vi "CRYGraph Set.vi"(9 "Title State":bool, 10 "Graph Property":T2, 11 "pGraph VI In":refnum<vi>) -> ()   [LabVIEW 2013]
uses:
  Control/CRYPolar Property.ctl
  Control/CRYTable Property.ctl
  Control/CRYGraph Property.ctl
  Control/CRYResult Property.ctl
panel:
  in  "Result Property":T1={"Show Limits"=FALSE, "Show Yield"=FALSE, "Pass/Fail"=FALSE, "Notation"=0, "Digits"=0, "Precision"=0, "Hide Traling Zeros"=FALSE, "Show vertical scroll bar"=FALSE, "Show horizontal scroll bar"=FALSE, "True"="NO ELECTRICAL SIGNAL DETECTED!\nCheck wiring and connections.", "False"="NO ELECTRICAL SIGNAL DETECTED!\nCheck wiring and connections.", "Font Size"=0, "Overall/Optional"=0} {"Precision" items=["Digits of precision", "Significant digits"]}
  in  "Table Property":T3 {"Precision" items=["Digits of precision", "Significant digits"]}
  in  "Polar Property":T4={"polar attributes"={"maximum"=2.0, "minimum"=0.0, "clip to min"=FALSE, "log"=FALSE, "grid color"=3381657, "plot color"=16711680, "fmt and prec"={"format"=enum."Decimal", "precision"=2}, "visible section"=4}, "Auto/Manual"=0, "Zero Adjust (deg)"=0, "Angle Increment (deg)"=0, "Mirror"=FALSE, "Auto Increment"=FALSE, "Total Rotatin (deg)"=0, "Discrete/Rannge"=0, "Show Name"=FALSE, "CurValues"=[], "CurIndex"=0, "CurColors"=[], "CurColors_Range"=[], "CurValues_Range"=[], "Pen"={"Width"=1, "Style"=enum."Solid"}, "BackgroundColor"=0} {"polar attributes"."minimum" format="%0.2f"; "polar attributes"."maximum" format="%0.2f"}
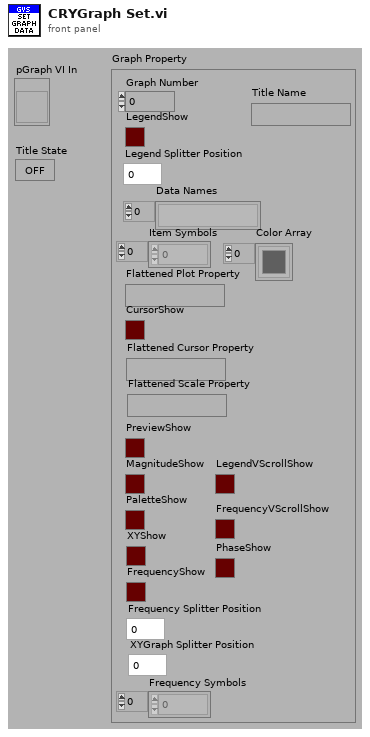
[diagram p1: front panel]
types:
  T1 = typedef "CRYResult Property.ctl" = cluster{"Show Limits":bool, "Show Yield":bool, "Pass/Fail":bool, "Notation":u16, "Digits":u16, "Precision":u16, "Hide Traling Zeros":bool, "Show vertical scroll bar":bool, "Show horizontal scroll bar":bool, "True":string, "False":string, "Font Size":u16, "Overall/Optional":u16}
  T2 = typedef "CRYGraph Property.ctl" = cluster{"LegendShow":bool, "Legend Splitter Position":dbl, "Data Names":string[], "Item Symbols":i32[], "Color Array":u32[], "Flattened Plot Property":string, "CursorShow":bool, "Flattened Cursor Property":string, "Graph Number":i32, "Flattened Scale Property":string, "PreviewShow":bool, "MagnitudeShow":bool, "PaletteShow":bool, "XYShow":bool, "FrequencyShow":bool, "Frequency Splitter Position":dbl, "XYGraph Splitter Position":dbl, "Frequency Symbols":i32[], "LegendVScrollShow":bool, "FrequencyVScrollShow":bool, "PhaseShow":bool, "Title Name":string}
  T3 = typedef "CRYTable Property.ctl" = cluster{"Reset All Columns":bool, "Transpose":bool, "Display Units":bool, "Notation":u16, "Digits":u16, "Precision":u16, "Hide Traling Zeros":bool, "Column Width":u16, "Row Header Width":u16, "Show vertical scroll bar":bool, "Show horizontal scroll bar":bool}
  T4 = typedef "CRYPolar Property.ctl" = cluster{"polar attributes":cluster{"maximum":dbl, "minimum":dbl, "clip to min":bool, "log":bool, "grid color":u32, "plot color":u32, "fmt and prec":cluster{"format":enum8{"Decimal", "Scientific", "Engineering", "Binary", "Octal", "Hex"}, "precision":u8}, "visible section":u16}, "Auto/Manual":u16, "Zero Adjust (deg)":i32, "Angle Increment (deg)":i32, "Mirror":bool, "Auto Increment":bool, "Total Rotatin (deg)":i32, "Discrete/Rannge":u16, "Show Name":bool, "CurValues":dbl[], "CurIndex":u16, "CurColors":u32[], "CurColors_Range":u32[], "CurValues_Range":dbl[], "Pen":cluster{"Width":u16, "Style":enum32{"Solid", "Dash", "Dot", "DashDot", "DashDotDot"}}, "BackgroundColor":u32}
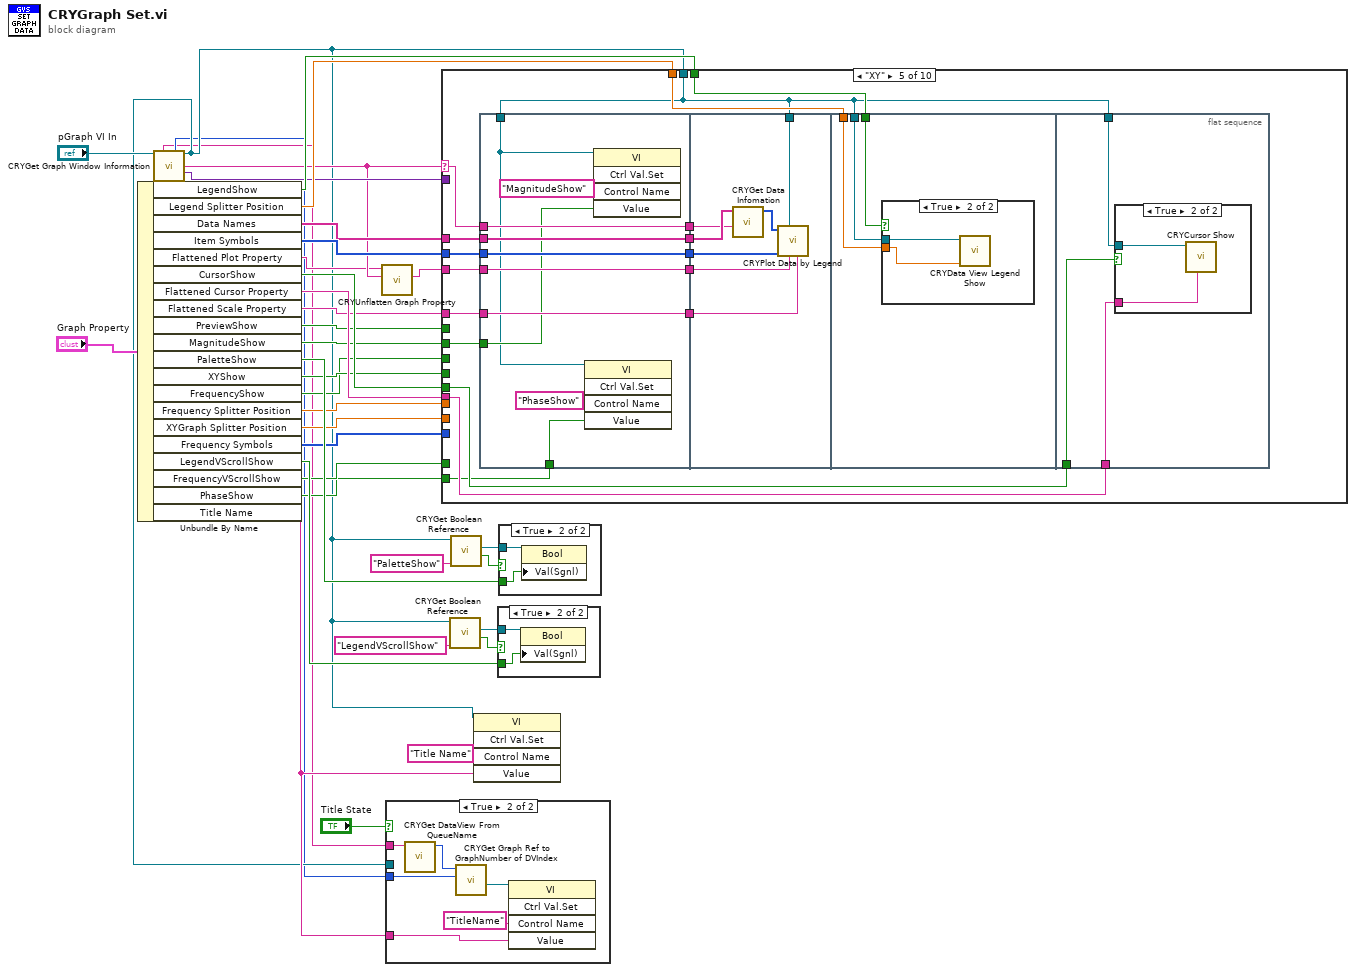
[diagram p0: block diagram]
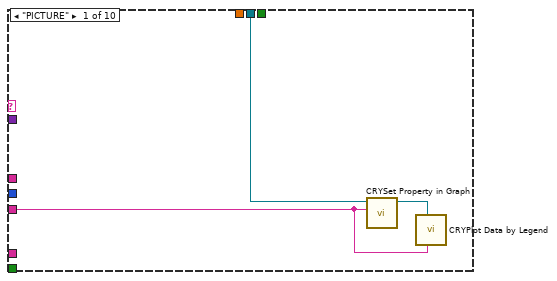
[diagram p5: hidden frame]
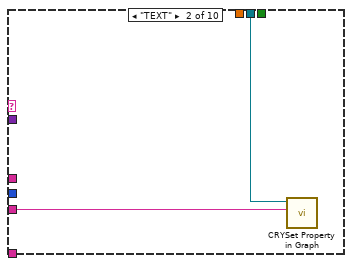
[diagram p6: hidden frame]
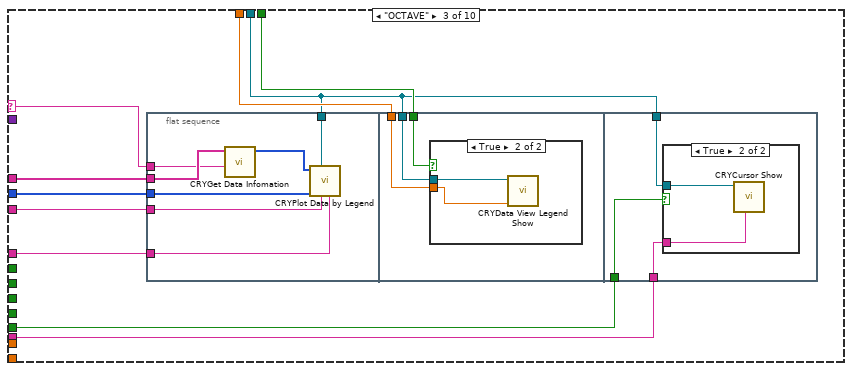
[diagram p7: hidden frame]
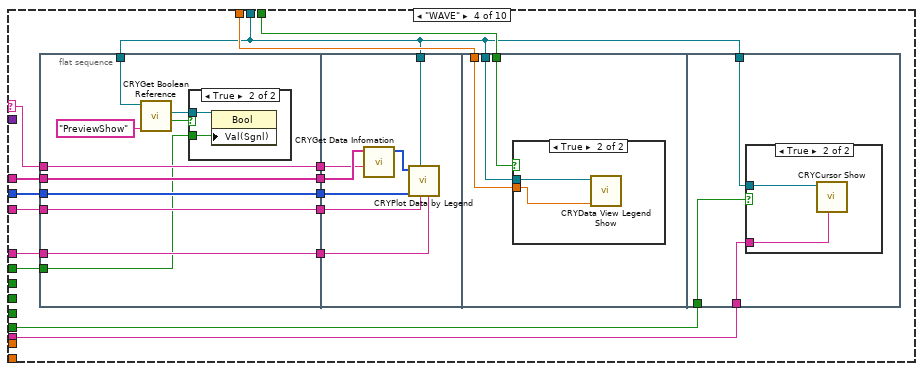
[diagram p10: hidden frame]
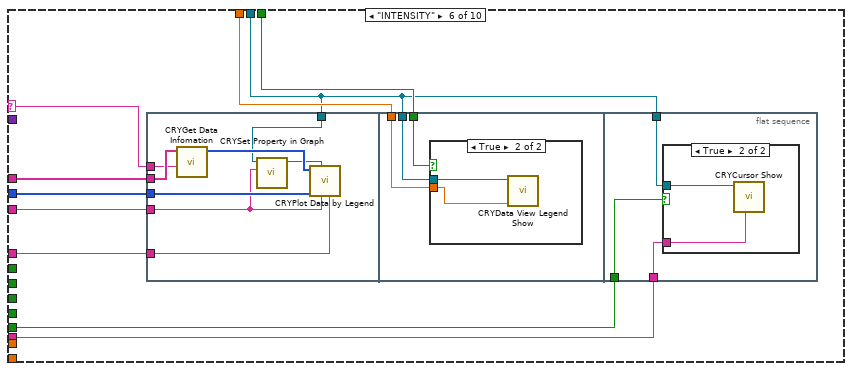
[diagram p16: hidden frame]
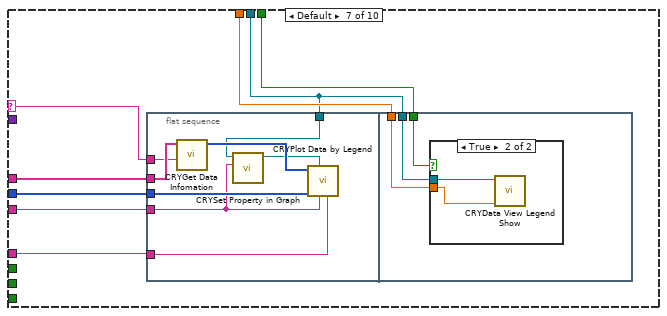
[diagram p19: hidden frame]
diagram:
  n1 = Unbundle By Name("Graph Property") -> ("LegendShow"=w31:bool, "Legend Splitter Position"=w32:dbl, "Data Names"=w33:string[], "Item Symbols"=w34:i32[], "Flattened Plot Property"=w14:string, "CursorShow"=w30:bool, "Flattened Cursor Property"=w29:string, "Flattened Scale Property"=w28:string, "PreviewShow"=w27:bool, "MagnitudeShow"=w26:bool, "PaletteShow"=w22:bool, "XYShow"=w21:bool, "FrequencyShow"=w17:bool, "Frequency Splitter Position"=w19:dbl, "XYGraph Splitter Position"=w18:dbl, "Frequency Symbols"=w20:i32[], "LegendVScrollShow"=w9:bool, "FrequencyVScrollShow"=w8:bool, "PhaseShow"=w7:bool, "Title Name"=w5:string)
  n2 = call "CRYGet Graph Window Information.vi"("pGraph VI In"="pGraph VI In") -> ("Queue Name Out"=w1:string, "Graph Number Out"=w2:i32, "pGraph VI Out"=w3:refnum<vi>, "Graph Type Out"=w15:string, "Graph Control Ref Out"=w16:variant)  [unwired: 4 in, 6 out]
  n3 = call "CRYUnflatten Graph Property.vi"("Cluster Name"=w15, "Flatten Graph Property"=w14) -> ("Flatten Graph Property Out"=w13:string)  [unwired: 7 in, 2 out]
  n4 = case shown="True" "Title State" {
    tunnel: w5 -> [_ w41]
    tunnel: w3 -> [_ _]
    tunnel: w2 -> [_ w39]
    tunnel: w1 -> [_ w40]
    frame False {
    }
    frame True {
      n5 = call "CRYGet DataView From QueueName.vi"("DataView QueueName"=w40) -> ("DataView Arrary Idx out"=w38:i32)  [unwired: 8 in, 2 out]
      n6 = call "CRYGet Graph Ref to GraphNumber of DVIndex.vi"("Graph Number"=w39, "DV Array index"=w38) -> ("Frame VIRef"=w37:refnum<vi>)  [unwired: 7 in, 2 out]
      n7 = invoke class="VI" method="Ctrl Val.Set"(reference=w37, "Control Name"="TitleName", "Value"=w41) -> ()  [unwired: 2 in, 5 out]
    }
  }
  n8 = case shown="\"XY\"" w15 {
    selector: w15 -> [_ _ w52 w85 w131 w168 w193 w236 w279 w301]
    tunnel: w34 -> [_ _ w57 w90 w136 w173 w199 w240 _ _]
    tunnel: w33 -> [_ _ w56 w89 w135 w172 w198 w239 w278 w300]
    tunnel: w28 -> [_ _ w48 w82 w128 w164 w197 w238 _ _]
    tunnel: w13 -> [w44 w47 w55 w88 w134 w171 w196 w237 w276 w298]
    tunnel: w32 -> [_ _ w54 w87 w133 w170 w195 w229 _ _]
    tunnel: w3 -> [w45 w46 w49 w76 w122 w165 w192 w213 w277 w299]
    tunnel: w31 -> [_ _ w53 w86 w132 w169 w194 w230 _ _]
    tunnel: w30 -> [_ _ w51 w84 w130 w167 _ _ _ _]
    tunnel: w29 -> [_ _ w50 w83 w129 w166 _ _ _ _]
    tunnel: w27 -> [_ _ _ w75 _ _ _ _ _ _]
    tunnel: w26 -> [_ _ _ _ w121 _ _ _ _ _]
    tunnel: w21 -> [_ _ _ _ _ _ _ w233 _ _]
    tunnel: w20 -> [_ _ _ _ _ _ _ w235 _ _]
    tunnel: w19 -> [_ _ _ _ _ _ _ w234 _ _]
    tunnel: w18 -> [_ _ _ _ _ _ _ w232 _ _]
    tunnel: w17 -> [_ _ _ _ _ _ _ w231 _ _]
    tunnel: w16 -> [_ _ _ _ _ _ _ _ w273 w295]
    tunnel: w8 -> [_ _ _ _ _ _ _ w214 _ _]
    tunnel: w7 -> [_ _ _ _ w120 _ _ _ _ _]
    frame "PICTURE" {
      n9 = call "CRYSet Property in Graph.vi"("Flatten Data String"=w44, "pGraph VI"=w45) -> ("pGraph VI Out"=w43:refnum<vi>)  [unwired: 9 in]
      n10 = call "CRYPlot Data by Legend.vi"("Flattened Plot Property"=w44, "pGraph VI"=w43) -> ()  [unwired: 7 in, 3 out]
    }
    frame "TEXT" {
      n11 = call "CRYSet Property in Graph.vi"("Flatten Data String"=w47, "pGraph VI"=w46) -> ()  [unwired: 9 in, 1 out]
    }
    frame "OCTAVE" {
      n12 = flat-sequence {
        tunnel: w52 -> [w63]
        tunnel: w56 -> [w64]
        tunnel: w57 -> [w60]
        tunnel: w48 -> [w61]
        tunnel: w55 -> [w58]
        tunnel: w49 -> [w62]
        tunnel: w54 -> [w67]
        tunnel: w49 -> [w66]
        tunnel: w53 -> [w65]
        tunnel: w51 -> [w72]
        tunnel: w50 -> [w71]
        tunnel: w49 -> [w70]
        frame #0 {
          n13 = call "CRYGet Data Infomation.vi"("Graph Type"=w63, "Data Names"=w64) -> ("Rows"=w59:i32[])  [unwired: 1 in, 8 out]
          n14 = call "CRYPlot Data by Legend.vi"("Flattened Scale Property"=w61, "Flattened Plot Property"=w58, "pGraph VI"=w62, "Legend Symbols"=w60, "Rows"=w59) -> ()  [unwired: 4 in, 3 out]
        }
        frame #1 {
          n15 = case shown="True" w65 {
            tunnel: w67 -> [_ w68]
            tunnel: w66 -> [_ w69]
            frame False {
            }
            frame True {
              n16 = call "CRYData View Legend Show.vi"("Legend Splitter Position"=w68, "pGraph VI"=w69) -> ()  [unwired: 2 in, 8 out]
            }
          }
        }
        frame #2 {
          n17 = case shown="True" w72 {
            tunnel: w70 -> [_ w74]
            tunnel: w71 -> [_ w73]
            frame False {
            }
            frame True {
              n18 = call "CRYCursor Show.vi"("Flattened Cursor Property"=w73, "pGraph VI"=w74) -> ()  [unwired: 10 in]
            }
          }
        }
      }
    }
    frame "WAVE" {
      n19 = flat-sequence {
        tunnel: w88 -> [w96]
        tunnel: w82 -> [w97]
        tunnel: w90 -> [w98]
        tunnel: w89 -> [w99]
        tunnel: w85 -> [w100]
        tunnel: [w100] -> w81
        tunnel: [w99] -> w80
        tunnel: [w98] -> w79
        tunnel: [w97] -> w78
        tunnel: [w96] -> w77
        tunnel: w76 -> [w91]
        tunnel: w75 -> [w92]
        tunnel: w76 -> [w107]
        tunnel: w81 -> [w108]
        tunnel: w80 -> [w109]
        tunnel: w79 -> [w105]
        tunnel: w78 -> [w106]
        tunnel: w77 -> [w103]
        tunnel: w87 -> [w112]
        tunnel: w76 -> [w111]
        tunnel: w86 -> [w110]
        tunnel: w84 -> [w117]
        tunnel: w83 -> [w116]
        tunnel: w76 -> [w115]
        frame #0 {
          n20 = call "CRYGet Boolean Reference.vi"("Label Name"="PreviewShow", "VI Refnum"=w91) -> ("Exist?"=w95:bool, "Boolean Ref"=w93:refnum<vi>)  [unwired: 7 in, 1 out]
          n21 = case shown="True" w95 {
            tunnel: w93 -> [_ w102]
            tunnel: w92 -> [_ w101]
            frame False {
            }
            frame True {
              n22 = property class="Bool"(reference=w102, "Val(Sgnl)"=w101) -> ()  [unwired: 1 in, 2 out]
            }
          }
        }
        frame #1 {
          n23 = call "CRYGet Data Infomation.vi"("Graph Type"=w108, "Data Names"=w109) -> ("Rows"=w104:i32[])  [unwired: 1 in, 8 out]
          n24 = call "CRYPlot Data by Legend.vi"("Flattened Scale Property"=w106, "Flattened Plot Property"=w103, "pGraph VI"=w107, "Legend Symbols"=w105, "Rows"=w104) -> ()  [unwired: 4 in, 3 out]
        }
        frame #2 {
          n25 = case shown="True" w110 {
            tunnel: w112 -> [_ w113]
            tunnel: w111 -> [_ w114]
            frame False {
            }
            frame True {
              n26 = call "CRYData View Legend Show.vi"("Legend Splitter Position"=w113, "pGraph VI"=w114) -> ()  [unwired: 2 in, 8 out]
            }
          }
        }
        frame #3 {
          n27 = case shown="True" w117 {
            tunnel: w115 -> [_ w119]
            tunnel: w116 -> [_ w118]
            frame False {
            }
            frame True {
              n28 = call "CRYCursor Show.vi"("Flattened Cursor Property"=w118, "pGraph VI"=w119) -> ()  [unwired: 10 in]
            }
          }
        }
      }
    }
    frame "XY" {
      n29 = flat-sequence {
        tunnel: w134 -> [w142]
        tunnel: w128 -> [w143]
        tunnel: w136 -> [w144]
        tunnel: w135 -> [w145]
        tunnel: w131 -> [w146]
        tunnel: [w146] -> w127
        tunnel: [w145] -> w126
        tunnel: [w144] -> w125
        tunnel: [w143] -> w124
        tunnel: [w142] -> w123
        tunnel: w122 -> [w138]
        tunnel: w121 -> [w140]
        tunnel: w120 -> [w137]
        tunnel: w122 -> [w151]
        tunnel: w127 -> [w152]
        tunnel: w126 -> [w153]
        tunnel: w125 -> [w149]
        tunnel: w124 -> [w150]
        tunnel: w123 -> [w147]
        tunnel: w133 -> [w156]
        tunnel: w122 -> [w155]
        tunnel: w132 -> [w154]
        tunnel: w130 -> [w161]
        tunnel: w129 -> [w160]
        tunnel: w122 -> [w159]
        frame #0 {
          n30 = invoke class="VI" method="Ctrl Val.Set"(reference=w138, "Control Name"="PhaseShow", "Value"=w137) -> ()  [unwired: 2 in, 5 out]
          n31 = invoke class="VI" method="Ctrl Val.Set"(reference=w138, "Control Name"="MagnitudeShow", "Value"=w140) -> ()  [unwired: 2 in, 5 out]
        }
        frame #1 {
          n32 = call "CRYGet Data Infomation.vi"("Graph Type"=w152, "Data Names"=w153) -> ("Rows"=w148:i32[])  [unwired: 1 in, 8 out]
          n33 = call "CRYPlot Data by Legend.vi"("Flattened Scale Property"=w150, "Flattened Plot Property"=w147, "pGraph VI"=w151, "Legend Symbols"=w149, "Rows"=w148) -> ()  [unwired: 4 in, 3 out]
        }
        frame #2 {
          n34 = case shown="True" w154 {
            tunnel: w156 -> [_ w157]
            tunnel: w155 -> [_ w158]
            frame False {
            }
            frame True {
              n35 = call "CRYData View Legend Show.vi"("Legend Splitter Position"=w157, "pGraph VI"=w158) -> ()  [unwired: 2 in, 8 out]
            }
          }
        }
        frame #3 {
          n36 = case shown="True" w161 {
            tunnel: w159 -> [_ w163]
            tunnel: w160 -> [_ w162]
            frame False {
            }
            frame True {
              n37 = call "CRYCursor Show.vi"("Flattened Cursor Property"=w162, "pGraph VI"=w163) -> ()  [unwired: 10 in]
            }
          }
        }
      }
    }
    frame "INTENSITY" {
      n38 = flat-sequence {
        tunnel: w168 -> [w180]
        tunnel: w172 -> [w181]
        tunnel: w173 -> [w178]
        tunnel: w164 -> [w179]
        tunnel: w171 -> [w176]
        tunnel: w165 -> [w174]
        tunnel: w170 -> [w184]
        tunnel: w165 -> [w183]
        tunnel: w169 -> [w182]
        tunnel: w167 -> [w189]
        tunnel: w166 -> [w188]
        tunnel: w165 -> [w187]
        frame #0 {
          n39 = call "CRYGet Data Infomation.vi"("Graph Type"=w180, "Data Names"=w181) -> ("Rows"=w177:i32[])  [unwired: 1 in, 8 out]
          n40 = call "CRYSet Property in Graph.vi"("Flatten Data String"=w176, "pGraph VI"=w174) -> ("pGraph VI Out"=w175:refnum<vi>)  [unwired: 9 in]
          n41 = call "CRYPlot Data by Legend.vi"("Flattened Scale Property"=w179, "Flattened Plot Property"=w176, "pGraph VI"=w175, "Legend Symbols"=w178, "Rows"=w177) -> ()  [unwired: 4 in, 3 out]
        }
        frame #1 {
          n42 = case shown="True" w182 {
            tunnel: w184 -> [_ w185]
            tunnel: w183 -> [_ w186]
            frame False {
            }
            frame True {
              n43 = call "CRYData View Legend Show.vi"("Legend Splitter Position"=w185, "pGraph VI"=w186) -> ()  [unwired: 2 in, 8 out]
            }
          }
        }
        frame #2 {
          n44 = case shown="True" w189 {
            tunnel: w187 -> [_ w191]
            tunnel: w188 -> [_ w190]
            frame False {
            }
            frame True {
              n45 = call "CRYCursor Show.vi"("Flattened Cursor Property"=w190, "pGraph VI"=w191) -> ()  [unwired: 10 in]
            }
          }
        }
      }
    }
    frame Default {
      n46 = flat-sequence {
        tunnel: w193 -> [w206]
        tunnel: w198 -> [w207]
        tunnel: w199 -> [w203]
        tunnel: w197 -> [w205]
        tunnel: w196 -> [w200]
        tunnel: w192 -> [w202]
        tunnel: w195 -> [w210]
        tunnel: w192 -> [w209]
        tunnel: w194 -> [w208]
        frame #0 {
          n47 = call "CRYGet Data Infomation.vi"("Graph Type"=w206, "Data Names"=w207) -> ("Rows"=w204:i32[])  [unwired: 1 in, 8 out]
          n48 = call "CRYSet Property in Graph.vi"("Flatten Data String"=w200, "pGraph VI"=w202) -> ("pGraph VI Out"=w201:refnum<vi>)  [unwired: 9 in]
          n49 = call "CRYPlot Data by Legend.vi"("Flattened Scale Property"=w205, "Flattened Plot Property"=w200, "pGraph VI"=w201, "Legend Symbols"=w203, "Rows"=w204) -> ()  [unwired: 4 in, 3 out]
        }
        frame #1 {
          n50 = case shown="True" w208 {
            tunnel: w210 -> [_ w211]
            tunnel: w209 -> [_ w212]
            frame False {
            }
            frame True {
              n51 = call "CRYData View Legend Show.vi"("Legend Splitter Position"=w211, "pGraph VI"=w212) -> ()  [unwired: 2 in, 8 out]
            }
          }
        }
      }
    }
    frame "POLAR" {
      n52 = flat-sequence {
        tunnel: w236 -> [w250]
        tunnel: w239 -> [w251]
        tunnel: w240 -> [w244]
        tunnel: w238 -> [w249]
        tunnel: w237 -> [w246]
        tunnel: w213 -> [w247]
        tunnel: w235 -> [w245]
        tunnel: [w243] -> w222
        tunnel: w234 -> [w254]
        tunnel: w231 -> [w253]
        tunnel: w222 -> [w252]
        tunnel: [w252] -> w221
        tunnel: w233 -> [w257]
        tunnel: w232 -> [w256]
        tunnel: w221 -> [w255]
        tunnel: [w255] -> w220
        tunnel: [w255] -> w218
        tunnel: w230 -> [w262]
        tunnel: w229 -> [w261]
        tunnel: w220 -> [w260]
        tunnel: [w260] -> w219
        tunnel: w223 -> [w267]
        tunnel: w219 -> [w266]
        frame #0 {
          n53 = call "CRYGet Data Infomation.vi"("Graph Type"=w250, "Data Names"=w251) -> ("Rows"=w248:i32[])  [unwired: 1 in, 8 out]
          n54 = call "CRYSet Property in Graph.vi"("Flatten Data String"=w246, "pGraph VI"=w247) -> ("pGraph VI Out"=w243:refnum<vi>)  [unwired: 9 in]
          n55 = call "CRYPlot Data by Legend.vi"("Flattened Scale Property"=w249, "Frequency Symbols"=w245, "Flattened Plot Property"=w246, "pGraph VI"=w243, "Legend Symbols"=w244, "Rows"=w248) -> ()  [unwired: 3 in, 3 out]
        }
        frame #1 {
          n56 = call "CRYFrequency Show.vi"("Frequency Splitter Position"=w254, "FrequencyShow"=w253, "pGraph VI"=w252) -> ()  [unwired: 9 in]
        }
        frame #2 {
          n57 = case shown="True" w257 {
            tunnel: w256 -> [_ w259]
            tunnel: w255 -> [_ w258]
            frame False {
            }
            frame True {
              n58 = call "CRYXY Graph Show.vi"("Frequency Splitter Position"=w259, "pGraph VI"=w258) -> ()  [unwired: 9 in, 1 out]
            }
          }
        }
        frame #3 {
          n59 = case shown="True" w262 {
            tunnel: w260 -> [_ w264]
            tunnel: w261 -> [_ w263]
            frame False {
            }
            frame True {
              n60 = call "CRYData View Legend Show.vi"("Legend Splitter Position"=w263, "sOption"="Polar_XY_Legend", "pGraph VI"=w264) -> ()  [unwired: 9 in]
            }
          }
        }
        frame #4 {
          n61 = call "CRYGet String Reference.vi"("Label Name"="XYCursor", "VI Refnum"=w266) -> ("String Ref Out"=w272:refnum<vi>)  [unwired: 7 in, 2 out]
          n62 = Select(t="Discrete" ("Value (Signaling)"), s=w267, f="Range" ("Value (Signaling)")) -> (s? t:f=w268:string)
          n63 = property class="Str"(reference=w272, "Val(Sgnl)"=w268) -> ()  [unwired: 1 in, 2 out]
        }
      }
      n64 = invoke class="VI" method="Ctrl Val.Get"(reference=w218, "Control Name"="Polar Property") -> ("Get Control Value Variant"=w226:variant)  [unwired: 2 in, 3 out]
      n65 = call "CRYGet Boolean Reference.vi"("Label Name"="FrequencyVScrollShow", "VI Refnum"=w213) -> ("Exist?"=w217:bool, "Boolean Ref"=w215:refnum<vi>)  [unwired: 7 in, 1 out]
      n66 = case shown="True" w217 {
        tunnel: w215 -> [_ w242]
        tunnel: w214 -> [_ w241]
        frame False {
        }
        frame True {
          n67 = property class="Bool"(reference=w242, "Val(Sgnl)"=w241) -> ()  [unwired: 1 in, 2 out]
        }
      }
      n68 = Variant To Data(type="Polar Property", Variant=w226) -> (data=w225:T4)  [unwired: 1 in, 1 out]
      n69 = Unbundle By Name(w225) -> ("Discrete/Rannge"=w224:u16)
      n70 = Equal To 0?(x=w224) -> (x = 0?=w223:bool)
    }
    frame "RESULT" {
      n71 = flat-sequence {
        tunnel: w279 -> [w286]
        tunnel: w278 -> [w285]
        tunnel: w277 -> [w283]
        tunnel: w276 -> [w281]
        tunnel: [w281] -> w275
        tunnel: [w280] -> w274
        tunnel: w273 -> [w280]
        tunnel: w275 -> [w288]
        tunnel: w274 -> [w287]
        frame #0 {
          n72 = call "CRYGet Data Infomation.vi"("Graph Type"=w286, "Data Names"=w285) -> ("Rows"=w284:i32[])  [unwired: 1 in, 8 out]
          n73 = call "CRYSet Property in Graph.vi"("Flatten Data String"=w281, "pGraph VI"=w283) -> ("pGraph VI Out"=w282:refnum<vi>)  [unwired: 9 in]
          n74 = call "CRYPlot Data by Legend.vi"("Flattened Plot Property"=w281, "pGraph VI"=w282, "Rows"=w284) -> ()  [unwired: 6 in, 3 out]
        }
        frame #1 {
          w293 = refnum<vi> refnum  # MulticolumnListbox
          n75 = Unflatten From String(type="Result Property", binary string=w288) -> (value=w294:T1)  [unwired: 3 in, 2 out]
          n76 = Variant To Data(type=w293, Variant=w287) -> (data=w292:refnum<vi>)  [unwired: 1 in, 1 out]
          n77 = Unbundle By Name(w294) -> ("Show vertical scroll bar"=w291:bool, "Show horizontal scroll bar"=w290:bool)
          n78 = property class="MCListbox"(reference=w292, "VScrollVis"=w291, "HScrollVis"=w290) -> ()  [unwired: 1 in, 2 out]
        }
      }
    }
    frame "TABLE" {
      n79 = flat-sequence {
        tunnel: w301 -> [w310]
        tunnel: w300 -> [w309]
        tunnel: w299 -> [w305]
        tunnel: w298 -> [w303]
        tunnel: [w303] -> w297
        tunnel: [w302] -> w296
        tunnel: w295 -> [w302]
        tunnel: w297 -> [w317]
        tunnel: w296 -> [w314]
        frame #0 {
          n80 = call "CRYGet Data Infomation.vi"("Graph Type"=w310, "Data Names"=w309) -> ("Result Rows"=w306:i32[], "Value Rows"=w307:i32[], "Rows"=w308:i32[])  [unwired: 1 in, 6 out]
          n81 = call "CRYSet Property in Graph.vi"("Flatten Data String"=w303, "pGraph VI"=w305) -> ("pGraph VI Out"=w304:refnum<vi>)  [unwired: 9 in]
          n82 = call "CRYPlot Data by Legend.vi"("Flattened Plot Property"=w303, "pGraph VI"=w304, "Result Rows"=w306, "Value Rows"=w307, "Rows"=w308) -> ()  [unwired: 5 in, 2 out]
        }
        frame #1 {
          w315 = refnum<vi> refnum  # Table
          n83 = Unflatten From String(type="Table Property", binary string=w317) -> (value=w316:T3)  [unwired: 3 in, 2 out]
          n84 = Variant To Data(type=w315, Variant=w314) -> (data=w313:refnum<vi>)  [unwired: 1 in, 1 out]
          n85 = Unbundle By Name(w316) -> ("Show vertical scroll bar"=w312:bool, "Show horizontal scroll bar"=w311:bool)
          n86 = property class="Tbl"(reference=w313, "Vert Scrollbar"=w312, "Horiz Scrollbar"=w311) -> ()  [unwired: 1 in, 2 out]
        }
      }
    }
  }
  n87 = call "CRYGet Boolean Reference.vi"("Label Name"="LegendVScrollShow", "VI Refnum"=w3) -> ("Exist?"=w10:bool, "Boolean Ref"=w12:refnum<vi>)  [unwired: 7 in, 1 out]
  n88 = call "CRYGet Boolean Reference.vi"("Label Name"="PaletteShow", "VI Refnum"=w3) -> ("Exist?"=w25:bool, "Boolean Ref"=w23:refnum<vi>)  [unwired: 7 in, 1 out]
  n89 = invoke class="VI" method="Ctrl Val.Set"(reference=w3, "Control Name"="Title Name", "Value"=w5) -> ()  [unwired: 2 in, 5 out]
  n90 = case shown="True" w10 {
    tunnel: w12 -> [_ w320]
    tunnel: w9 -> [_ w319]
    frame False {
    }
    frame True {
      n91 = property class="Bool"(reference=w320, "Val(Sgnl)"=w319) -> ()  [unwired: 1 in, 2 out]
    }
  }
  n92 = case shown="True" w25 {
    tunnel: w23 -> [_ w322]
    tunnel: w22 -> [_ w321]
    frame False {
    }
    frame True {
      n93 = property class="Bool"(reference=w322, "Val(Sgnl)"=w321) -> ()  [unwired: 1 in, 2 out]
    }
  }
